vi "Stop Worker.vi"(8 "error in (no error)":errorcluster, 11 "BuildServer in":refnum<class "BuildServer.lvclass">) -> (0 "error out":errorcluster, 3 "BuildServer out":refnum<class "BuildServer.lvclass">)   [LabVIEW 2017, in "BuildServer.lvlib" / "BuildServer.lvclass"]
uses:
  BuildServer.lvclass
  BuildServer.lvclass/BuildServer.ctl
  Classes/Comm Interface/Comm Interface.lvclass
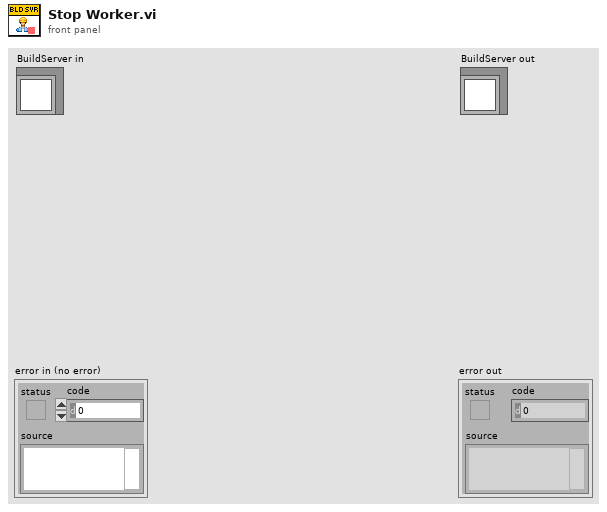
[diagram p1: front panel]
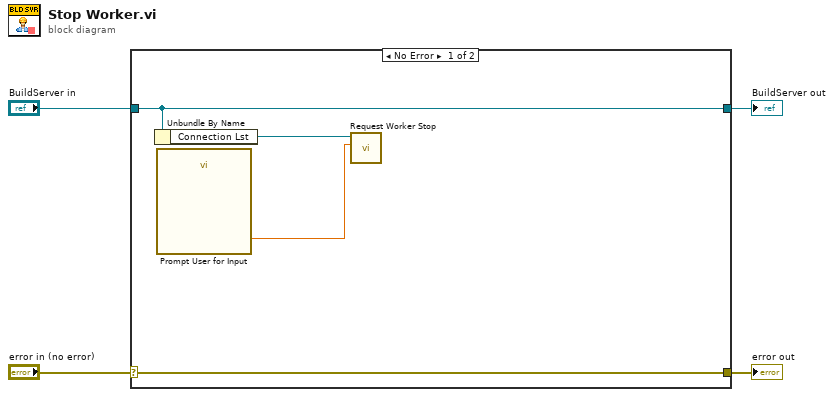
[diagram p0: block diagram]
diagram:
  n1 = case shown="No Error" "error in (no error)" {
    selector: "error in (no error)" -> [w8 w10]
    tunnel: [w8 w10] -> w3
    tunnel: [w7 w9] -> w1
    tunnel: "BuildServer in" -> [w7 w9]
    frame No Error {
      n2 = Unbundle By Name(w7) -> ("Connection Lst"=w6:refnum<class "Comm Interface.lvclass">)
      n3 = call "Prompt User for Input"() -> ("Worker Index"=w5:dbl)  [unwired: 17 in, 2 out]
      n4 = call "Request Worker Stop.vi"("index"=w5, "Comm Interface in"=w6) -> ()  [unwired: 8 in, 2 out]
    }
    frame Error {
    }
  }
  "error out" <- w3
  "BuildServer out" <- w1
